vi "Is Window Being Shown (class variable).vi"() -> ()   [LabVIEW 2023, in "Error Manager.lvlib" / "Error Display Window.lvclass"]
uses:
  Error Display Window.lvclass
panel:
  out "Is Window Being Shown?":bool
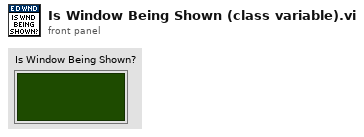
[diagram p1: front panel]
diagram:
